vi "Begin.vi"(8 "error in":errorcluster) -> (0 "error out":errorcluster)   [LabVIEW 2017]
doc: "Called before other user functions, this VI is expected to open initial I/O refnums, load in file data, and do all program initialization. Notice that the <B>error out</B> terminal is simply used for data flow. Wiring it to other structures or subVIs ensures that this VI runs first."
uses:
  <vilib>/Rock Robotics/WPI/DriverStation/WPI_DriverStationRobotMode2.ctl
  <vilib>/Rock Robotics/WPI/Joystick/WPI_JoystickDeviceEnum.ctl
  <vilib>/Rock Robotics/WPI/ThirdParty/Phoenix-LabVIEW/Motor Controller/Controls/CTRE_Phoenix_MotorControl_ControlMode.ctl
  <vilib>/Rock Robotics/WPI/ThirdParty/Phoenix-LabVIEW/Motor Controller/Controls/CTRE_Phoenix_MotorControl_NeutralMode.ctl
  <vilib>/Rock Robotics/WPI/ThirdParty/Phoenix-LabVIEW/Motor Controller/Controls/CTRE_Phoenix_MotorControl_FeedbackDevice.ctl
  <vilib>/Rock Robotics/SystemInterfaces/spilib/spi_bus.ctl
  <vilib>/Rock Robotics/WPI/Solenoid/WPI_SolenoidChannel.ctl
  <vilib>/Rock Robotics/SystemInterfaces/DIO/FPGA_DIOChannel.ctl
  Robot Global Data.vi
  <vilib>/Rock Robotics/Network Tables/NT Write Numeric Array.vi
  <vilib>/Rock Robotics/WPI/Utilities/WPI_GetSetVariantRefNum.vi
  <vilib>/Rock Robotics/WPI/Gyro/WPI_GyroXRS450_SPI_Open.vi
  <vilib>/Rock Robotics/WPI/Switch/WPI_SwitchOpenLimit.vi
  <vilib>/Rock Robotics/WPI/Solenoid/WPI_SolenoidOpenDouble.vi
  <vilib>/Rock Robotics/Network Tables/NT Write String Array.vi
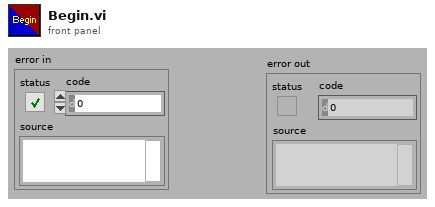
[diagram p1: front panel]
types:
  T1 = typedef "WPI_SolenoidChannel.ctl" = enum8{"Solenoid 0", "Solenoid 1", "Solenoid 2", "Solenoid 3", "Solenoid 4", "Solenoid 5", "Solenoid 6", "Solenoid 7", "Invalid"}
  T2 = typedef "FPGA_DIOChannel.ctl" = enum8{"DIO 0", "DIO 1", "DIO 2", "DIO 3", "DIO 4", "DIO 5", "DIO 6", "DIO 7", "DIO 8", "DIO 9", "DIO MXP 0", "DIO MXP 1", "DIO MXP 2", "DIO MXP 3", "DIO MXP 4", "DIO MXP 5", "DIO MXP 6", "DIO MXP 7", "DIO MXP 8", "DIO MXP 9", "DIO MXP 10", "DIO MXP 11", "DIO MXP 12", "DIO MXP 13", "DIO MXP 14", "DIO MXP 15", "SPI Port CS1", "SPI Port CS2", "SPI Port CS3", "SPI Port MISO", "SPI Port MOSI", "Invalid"}
  T3 = typedef "spi_bus.ctl" = enum16{"SPI On-Board, CS0", "SPI On-Board, CS1", "SPI On-Board, CS2", "SPI On-Board, CS3", "SPI MXP", "Invalid"}
  T4 = typedef "CTRE_Phoenix_MotorControl_FeedbackDevice.ctl" = i8
  T5 = typedef "CTRE_Phoenix_MotorControl_NeutralMode.ctl" = enum8{"EEPROMSetting", "Override to Coast", "Override to Brake"}
  T6 = typedef "CTRE_Phoenix_MotorControl_ControlMode.ctl" = u16
  T7 = typedef "WPI_JoystickDeviceEnum.ctl" = enum16{"USB 0", "USB 1", "USB 2", "USB 3", "USB 4", "USB 5"}
  T8 = typedef "WPI_DriverStationRobotMode2.ctl" = enum16{"Autonomous Disabled", "Autonomous Enabled", "Teleop Disabled", "Teleop Enabled", "Disconnected", "Finish", "Test Disabled", "Test Enabled", "Emergency Stopped"}
  T9 = typedef "WPI_SolenoidDevRef.ctl" = cluster{"DevStatus":errorcluster, "Pneumatics Control Module":u8, "Forward Solenoid Channel":T1, "Reverse Solenoid Channel":T1}
  T10 = typedef "WPI_JoystickDevRef.ctl" = cluster{"Device":T7}
  T11 = typedef "WPI_SwitchDevRef.ctl" = cluster{"DevStatus":errorcluster, "DIO Channel":T2, "CntIndex":T12, "Normally Closed":bool}
  T12 = typedef "FPGA_CounterCtrSystemIndex.ctl" = enum8{"Ctr 0", "Ctr 1", "Ctr 2", "Ctr 3", "Ctr 4", "Ctr 5", "Ctr 6", "Ctr 7", "Invalid"}
  T13 = typedef "WPI_MotorControlDeviceRef.ctl" = cluster{"DeviceStatus":errorcluster, "Type":T14, "PWM":cluster{"PWM Channel":T15, "DeadBand":T16}, "CAN":cluster{"Device Number":u8, "SetOutput VI Ref":variant, "GetOutput VI Ref":variant, "Enable VI Ref":variant, "Disable VI Ref":variant, "Data":variant}, "Invert":bool, "DIO PWM":cluster{"PWM \"Enable\" Channel":T15, "DIOChannel":T2, "PWM Rate":dbl}}
  T14 = typedef "WPI_MotorControlType.ctl" = enum16{"PWM", "CAN", "DIO PWM"}
  T15 = typedef "FPGA_DIOPWMChannel.ctl" = enum8{"PWM 0", "PWM 1", "PWM 2", "PWM 3", "PWM 4", "PWM 5", "PWM 6", "PWM 7", "PWM 8", "PWM 9", "PWM MXP 0", "PWM MXP 1", "PWM MXP 2", "PWM MXP 3", "PWM MXP 4", "PWM MXP 5", "PWM MXP 6", "PWM MXP 7", "PWM MXP 8", "PWM MXP 9", "Invalid"}
  T16 = typedef "WPI_PWMDeadband.ctl" = cluster{"Name":string, "maxPositivePwm":i32, "minPositivePwm":i32, "centerPwm":i32, "maxNegativePwm":i32, "minNegativePwm":i32, "angularRange":u16}
  T17 = typedef "WPI_GyroDevRef.ctl" = cluster{"DevStatus":errorcluster, "Analog Channel":T18, "Gain (VoltsPerDegree/Second)":dbl, "Gyro Type":enum16{"Analog", "XRS450"}, "Handle":i32, "SPI Bus":T3, "Device Found":bool, "Sample Rate":dbl, "Calibrate On Open":bool, "Offset":dbl}
  T18 = typedef "FPGA_AIChannel.ctl" = enum8{"AI 0", "AI 1", "AI 2", "AI 3", "AI MXP 0", "AI MXP 1", "AI MXP 2", "AI MXP 3", "Invalid"}
  T19 = typedef "WPI_CompressorDevRef.ctl" = cluster{"DevStatus":errorcluster, "Pneumatics Control Module":u8}
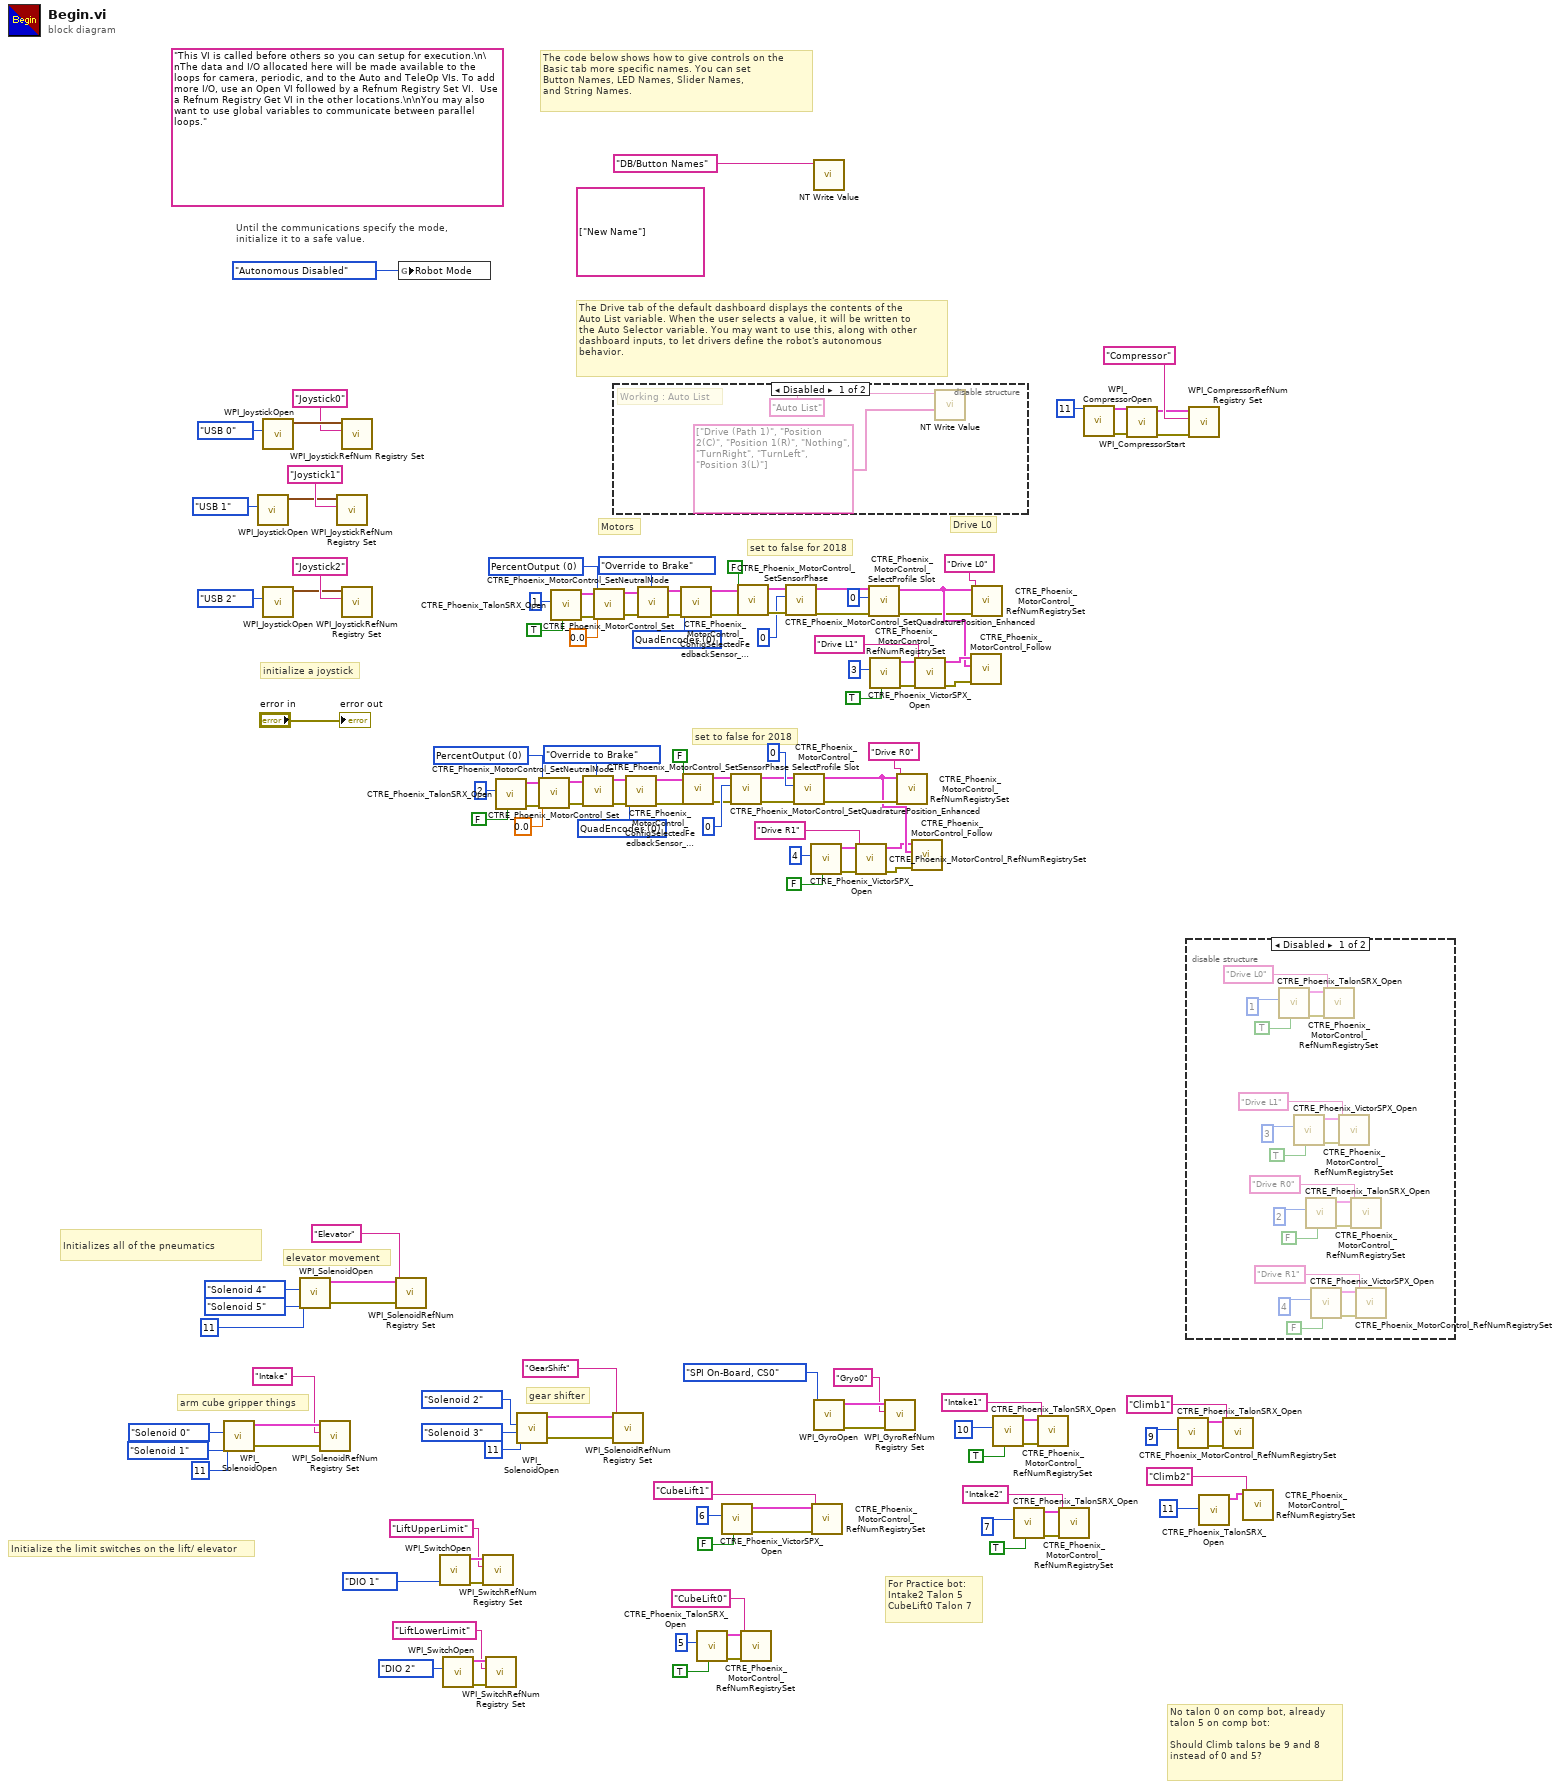
[diagram p0: block diagram]
diagram:
  w87 = T4 0 items=["None"=-1, "QuadEncoder"=0, "Analog"=2, "Tachometer"=4, "Pulse Width Encoded Position"=8, "Sensor Sum (S0 + S1)"=9, "Sensor Difference (D0 - D1)"=10, "Remote Source 0"=11, "Remote Source 1"=12, "Software Emulated"=15] ("Feedback Device")
  w82 = T6 0 items=["PercentOutput"=0, "Position"=1, "Velocity"=2, "Current"=3, "Follower"=5, "MotionProfile"=6, "MotionMagic"=7, "MotionMagicArc"=8, "MotionProfileArc"=10, "Disabled"=15] ("Control Mode")
  w106 = T4 0 items=["None"=-1, "QuadEncoder"=0, "Analog"=2, "Tachometer"=4, "Pulse Width Encoded Position"=8, "Sensor Sum (S0 + S1)"=9, "Sensor Difference (D0 - D1)"=10, "Remote Source 0"=11, "Remote Source 1"=12, "Software Emulated"=15] ("Feedback Device")
  w111 = T6 0 items=["PercentOutput"=0, "Position"=1, "Velocity"=2, "Current"=3, "Follower"=5, "MotionProfile"=6, "MotionMagic"=7, "MotionMagicArc"=8, "MotionProfileArc"=10, "Disabled"=15] ("Control Mode")
  (unwired) string[] ["New Name"]
  (unwired) "This VI is called before others so you can setup for execution.\n\nThe data and I/O allocated here will be made available to the loops for camera, periodic, and to the Auto and TeleOp VIs. To add more I/O, use an Open VI followed by a Refnum Registry Set VI.  Use a Refnum Registry Get VI in the other locations.\n\nYou may also want to use global variables to communicate between parallel loops."
  # "No talon 0 on comp bot, already\ntalon 5 on comp bot:\n\nShould Climb talons be 9 and 8\ninstead of 0 and 5?"
  # "gear shifter"
  # "arm cube gripper things"
  # "elevator movement"
  # "Initialize the limit switches on the lift/ elevator"
  # "Initializes all of the pneumatics"
  # "For Practice bot:\nIntake2 Talon 5\nCubeLift0 Talon 7"
  # "set to false for 2018"
  # "set to false for 2018"
  # "Drive L0"
  # "Motors"
  # "The Drive tab of the default dashboard displays the contents of the\nAuto List variable. When the user selects a value, it will be written to\nthe Auto Selector variable. You may want to use this, along with other\ndashboard inputs, to let drivers define the robot's autonomous\nbehavior."
  # "The code below shows how to give controls on the\nBasic tab more specific names. You can set\nButton Names, LED Names, Slider Names,\nand String Names."
  # "initialize a joystick"
  # "Until the communications specify the mode,\ninitialize it to a safe value."
  n1 = call-poly <vilib>:"WPI_SolenoidOpen.vi"("Reverse Solenoid Channel"=WPI_SolenoidChannel."Solenoid 1", "Forward Solenoid Channel"=WPI_SolenoidChannel."Solenoid 0", "Pneumatics Control Module (0)"=u8 11) -> ("error out"=w24:errorcluster, "SolenoidDevRef"=w23:T9)  [unwired: 7 in]
  n2 = call <vilib>:"WPI_JoystickOpen.vi"("JoystickDevice"=WPI_JoystickDeviceEnum."USB 1") -> ("JoystickDevRef"=w135:T10)  [unwired: 10 in]
  n3 = call <vilib>:"WPI_JoystickOpen.vi"("JoystickDevice"=WPI_JoystickDeviceEnum."USB 0") -> ("JoystickDevRef"=w130:T10)  [unwired: 10 in]
  n4 = call <vilib>:"WPI_JoystickOpen.vi"("JoystickDevice"=WPI_JoystickDeviceEnum."USB 2") -> ("JoystickDevRef"=w127:T10)  [unwired: 10 in]
  n5 = call-poly <vilib>:"WPI_SolenoidOpen.vi"("Reverse Solenoid Channel"=WPI_SolenoidChannel."Solenoid 5", "Forward Solenoid Channel"=WPI_SolenoidChannel."Solenoid 4", "Pneumatics Control Module (0)"=u8 11) -> ("error out"=w32:errorcluster, "SolenoidDevRef"=w31:T9)  [unwired: 7 in]
  n6 = call <vilib>:"WPI_SolenoidRefNum Registry Set.vi"("error in (no error)"=w24, "refnum name"="Intake", "SolenoidDevRef"=w23) -> ()  [unwired: 7 in, 2 out]
  n7 = call <vilib>:"WPI_JoystickRefNum Registry Set.vi"("refnum name"="Joystick1", "JoystickDevRef"=w135) -> ()  [unwired: 8 in, 2 out]
  n8 = call <vilib>:"WPI_JoystickRefNum Registry Set.vi"("refnum name"="Joystick0", "JoystickDevRef"=w130) -> ()  [unwired: 8 in, 2 out]
  n9 = call <vilib>:"WPI_JoystickRefNum Registry Set.vi"("refnum name"="Joystick2", "JoystickDevRef"=w127) -> ()  [unwired: 8 in, 2 out]
  n10 = call <vilib>:"WPI_SolenoidRefNum Registry Set.vi"("error in (no error)"=w32, "refnum name"="Elevator", "SolenoidDevRef"=w31) -> ()  [unwired: 7 in, 2 out]
  n11 = global write "Robot Global Data.vi" "Robot Mode"(WPI_DriverStationRobotMode2."Autonomous Disabled" ("Robot Mode")) -> ()
  n12 = call-poly <vilib>:"WPI_SwitchOpen.vi"("DIO Channel"=FPGA_DIOChannel."DIO 1") -> ("error out"=w20:errorcluster, "SwitchDevRef"=w19:T11)  [unwired: 9 in]
  n13 = call-poly <vilib>:"WPI_SwitchOpen.vi"("DIO Channel"=FPGA_DIOChannel."DIO 2") -> ("error out"=w17:errorcluster, "SwitchDevRef"=w16:T11)  [unwired: 9 in]
  n14 = call <vilib>:"WPI_SwitchRefNum Registry Set.vi"("error in (no error)"=w20, "refnum name"="LiftUpperLimit", "SwitchDevRef"=w19) -> ()  [unwired: 7 in, 2 out]
  n15 = call <vilib>:"WPI_SwitchRefNum Registry Set.vi"("error in (no error)"=w17, "refnum name"="LiftLowerLimit", "SwitchDevRef"=w16) -> ()  [unwired: 7 in, 2 out]
  n16 = call "CTRE_Phoenix_TalonSRX_Open.vi"("Invert"=FALSE, "Device Number"=u8 2) -> ("error out"=w79:errorcluster, "CAN Talon SRX Ref"=w78:T13)  [unwired: 8 in]
  n17 = call-poly <vilib>:"WPI_SolenoidOpen.vi"("Reverse Solenoid Channel"=WPI_SolenoidChannel."Solenoid 3", "Forward Solenoid Channel"=WPI_SolenoidChannel."Solenoid 2", "Pneumatics Control Module (0)"=u8 11) -> ("error out"=w25:errorcluster, "SolenoidDevRef"=w26:T9)  [unwired: 7 in]
  n18 = call <vilib>:"CTRE_Phoenix_MotorControl_Set.vi"("error in (no error)"=w79, "Output"=0.0, "Control Mode"=w82, "PhoenixMotorControlDevRef"=w78) -> ("error out"=w81:errorcluster, "PhoenixMotorControlDevRef"=w80:T13)  [unwired: 6 in]
  n19 = call "CTRE_Phoenix_TalonSRX_Open.vi"("Invert"=TRUE, "Device Number"=u8 1) -> ("error out"=w114:errorcluster, "CAN Talon SRX Ref"=w115:T13)  [unwired: 8 in]
  n20 = call <vilib>:"CTRE_Phoenix_MotorControl_SetNeutralMode.vi"("error in (no error)"=w81, "Motor Control Neutral Mode"=CTRE_Phoenix_MotorControl_NeutralMode."Override to Brake", "PhoenixMotorControlDevRef"=w80) -> ("error out"=w85:errorcluster, "PhoenixMotorControlDevRef"=w86:T13)  [unwired: 7 in]
  n21 = call <vilib>:"CTRE_Phoenix_MotorControl_Set.vi"("error in (no error)"=w114, "Output"=0.0, "Control Mode"=w111, "PhoenixMotorControlDevRef"=w115) -> ("error out"=w112:errorcluster, "PhoenixMotorControlDevRef"=w113:T13)  [unwired: 6 in]
  n22 = call <vilib>:"WPI_SolenoidRefNum Registry Set.vi"("error in (no error)"=w25, "refnum name"="GearShift", "SolenoidDevRef"=w26) -> ()  [unwired: 7 in, 2 out]
  n23 = disable-structure shown="Disabled" {
    frame Disabled {
      # "Working : Auto List"
      n24 = call-poly <vilib>:"NT Write Value.vi"("String Array"=string[] ["Drive (Path 1)", "Position 2(C)", "Position 1(R)", "Nothing", "TurnRight", "TurnLeft", "Position 3(L)"], "Name"="Auto List") -> ()  [unwired: 9 in, 1 out]
    }
    frame Enabled {
    }
  }
  n25 = call <vilib>:"CTRE_Phoenix_MotorControl_ConfigSelectedFeedbackSensor_Enhanced.vi"("error in (no error)"=w85, "Feedback Device"=w87, "PhoenixMotorControlDevRef"=w86) -> ("error out"=w89:errorcluster, "PhoenixMotorControlDevRef"=w88:T13)  [unwired: 7 in]
  n26 = call <vilib>:"CTRE_Phoenix_MotorControl_SetNeutralMode.vi"("error in (no error)"=w112, "Motor Control Neutral Mode"=CTRE_Phoenix_MotorControl_NeutralMode."Override to Brake", "PhoenixMotorControlDevRef"=w113) -> ("error out"=w108:errorcluster, "PhoenixMotorControlDevRef"=w107:T13)  [unwired: 7 in]
  n27 = call <vilib>:"CTRE_Phoenix_MotorControl_ConfigSelectedFeedbackSensor_Enhanced.vi"("error in (no error)"=w108, "Feedback Device"=w106, "PhoenixMotorControlDevRef"=w107) -> ("error out"=w104:errorcluster, "PhoenixMotorControlDevRef"=w105:T13)  [unwired: 7 in]
  n28 = call <vilib>:"CTRE_Phoenix_MotorControl_SetSensorPhase.vi"("error in (no error)"=w89, "PhaseSensor"=FALSE, "PhoenixMotorControlDevRef"=w88) -> ("error out"=w91:errorcluster, "PhoenixMotorControlDevRef"=w92:T13)  [unwired: 7 in]
  n29 = call "CTRE_Phoenix_TalonSRX_Open.vi"("Invert"=TRUE, "Device Number"=u8 5) -> ("error out"=w44:errorcluster, "CAN Talon SRX Ref"=w43:T13)  [unwired: 8 in]
  n30 = call <vilib>:"CTRE_Phoenix_VictorSPX_Open.vi"("Invert"=FALSE, "Device Number"=u8 6) -> ("error out"=w47:errorcluster, "CAN Talon SRX Ref"=w46:T13)  [unwired: 8 in]
  n31 = call <vilib>:"CTRE_Phoenix_MotorControl_SetQuadraturePosition_Enhanced.vi"("error in (no error)"=w91, "New Position"=0, "PhoenixMotorControlDevRef"=w92) -> ("error out"=w3:errorcluster, "PhoenixMotorControlDevRef"=w4:T13)  [unwired: 7 in]
  n32 = call <vilib>:"CTRE_Phoenix_MotorControl_SetSensorPhase.vi"("error in (no error)"=w104, "PhaseSensor"=FALSE, "PhoenixMotorControlDevRef"=w105) -> ("error out"=w102:errorcluster, "PhoenixMotorControlDevRef"=w101:T13)  [unwired: 7 in]
  n33 = call <vilib>:"CTRE_Phoenix_MotorControl_RefNumRegistrySet.vi"("error in (no error)"=w44, "refnum name"="CubeLift0", "PhoenixMotorControlDevRef"=w43) -> ()  [unwired: 7 in, 2 out]
  n34 = call <vilib>:"CTRE_Phoenix_MotorControl_SetQuadraturePosition_Enhanced.vi"("error in (no error)"=w102, "New Position"=0, "PhoenixMotorControlDevRef"=w101) -> ("error out"=w5:errorcluster, "PhoenixMotorControlDevRef"=w6:T13)  [unwired: 7 in]
  n35 = call <vilib>:"CTRE_Phoenix_MotorControl_SelectProfile Slot.vi"("error in (no error)"=w3, "slotIdx"=0, "PhoenixMotorControlDevRef"=w4) -> ("error out"=w95:errorcluster, "PhoenixMotorControlDevRef"=w94:T13)  [unwired: 7 in]
  n36 = call <vilib>:"CTRE_Phoenix_VictorSPX_Open.vi"("Invert"=FALSE, "Device Number"=u8 4) -> ("error out"=w71:errorcluster, "CAN Talon SRX Ref"=w72:T13)  [unwired: 8 in]
  n37 = call <vilib>:"CTRE_Phoenix_MotorControl_RefNumRegistrySet.vi"("error in (no error)"=w47, "refnum name"="CubeLift1", "PhoenixMotorControlDevRef"=w46) -> ()  [unwired: 7 in, 2 out]
  n38 = call-poly <vilib>:"NT Write Value.vi"("Name"="DB/Button Names") -> ()  [unwired: 10 in, 1 out]
  n39 = call-poly <vilib>:"WPI_GyroOpen.vi"("SPI Bus"=spi_bus."SPI On-Board, CS0") -> ("error out"=w39:errorcluster, "GyroDevRef"=w40:T17)  [unwired: 8 in, 1 out]
  n40 = call <vilib>:"CTRE_Phoenix_MotorControl_RefNumRegistrySet.vi"("error in (no error)"=w71, "refnum name"="Drive R1", "PhoenixMotorControlDevRef"=w72) -> ("error out"=w74:errorcluster, "PhoenixMotorControlDevRef"=w75:T13)  [unwired: 7 in]
  n41 = call <vilib>:"CTRE_Phoenix_MotorControl_SelectProfile Slot.vi"("error in (no error)"=w5, "slotIdx"=0, "PhoenixMotorControlDevRef"=w6) -> ("error out"=w98:errorcluster, "PhoenixMotorControlDevRef"=w99:T13)  [unwired: 7 in]
  n42 = call <vilib>:"CTRE_Phoenix_VictorSPX_Open.vi"("Invert"=TRUE, "Device Number"=u8 3) -> ("error out"=w122:errorcluster, "CAN Talon SRX Ref"=w121:T13)  [unwired: 8 in]
  n43 = call <vilib>:"WPI_GyroRefNum Registry Set.vi"("error in (no error)"=w39, "refnum name"="Gryo0", "GyroDevRef"=w40) -> ()  [unwired: 7 in, 2 out]
  n44 = call <vilib>:"CTRE_Phoenix_MotorControl_RefNumRegistrySet.vi"("error in (no error)"=w95, "refnum name"="Drive R0", "PhoenixMotorControlDevRef"=w94) -> ()  [unwired: 7 in, 2 out]
  n45 = call <vilib>:"CTRE_Phoenix_MotorControl_Follow.vi"("error in (no error)"=w74, "Master Controller to Follow"=w94, "PhoenixMotorControlDevRef"=w75) -> ()  [unwired: 7 in, 2 out]
  n46 = call <vilib>:"CTRE_Phoenix_MotorControl_RefNumRegistrySet.vi"("error in (no error)"=w122, "refnum name"="Drive L1", "PhoenixMotorControlDevRef"=w121) -> ("error out"=w119:errorcluster, "PhoenixMotorControlDevRef"=w118:T13)  [unwired: 7 in]
  n47 = call <vilib>:"CTRE_Phoenix_MotorControl_Follow.vi"("error in (no error)"=w119, "Master Controller to Follow"=w99, "PhoenixMotorControlDevRef"=w118) -> ()  [unwired: 7 in, 2 out]
  n48 = call <vilib>:"CTRE_Phoenix_MotorControl_RefNumRegistrySet.vi"("error in (no error)"=w98, "refnum name"="Drive L0", "PhoenixMotorControlDevRef"=w99) -> ()  [unwired: 7 in, 2 out]
  n49 = call "CTRE_Phoenix_TalonSRX_Open.vi"("Invert"=TRUE, "Device Number"=u8 10) -> ("error out"=w56:errorcluster, "CAN Talon SRX Ref"=w55:T13)  [unwired: 8 in]
  n50 = call "CTRE_Phoenix_TalonSRX_Open.vi"("Invert"=TRUE, "Device Number"=u8 7) -> ("error out"=w52:errorcluster, "CAN Talon SRX Ref"=w51:T13)  [unwired: 8 in]
  n51 = call <vilib>:"CTRE_Phoenix_MotorControl_RefNumRegistrySet.vi"("error in (no error)"=w56, "refnum name"="Intake1", "PhoenixMotorControlDevRef"=w55) -> ()  [unwired: 7 in, 2 out]
  n52 = call <vilib>:"CTRE_Phoenix_MotorControl_RefNumRegistrySet.vi"("error in (no error)"=w52, "refnum name"="Intake2", "PhoenixMotorControlDevRef"=w51) -> ()  [unwired: 7 in, 2 out]
  n53 = call <vilib>:"WPI_CompressorOpen.vi"("Pneumatics Control Module (0)"=u8 11) -> ("CompressorDevRef"=w66:T19, "error out"=w65:errorcluster)  [unwired: 13 in]
  n54 = call <vilib>:"WPI_CompressorStart.vi"("error in (no error)"=w65, "CompressorDevRef"=w66) -> ("error out"=w63:errorcluster, "CompressorDevRef"=w64:T19)  [unwired: 8 in]
  n55 = call "CTRE_Phoenix_TalonSRX_Open.vi"("Device Number"=u8 9) -> ("error out"=w61:errorcluster, "CAN Talon SRX Ref"=w60:T13)  [unwired: 9 in]
  n56 = disable-structure shown="Disabled" {
    frame Disabled {
      n57 = call "CTRE_Phoenix_TalonSRX_Open.vi"("Invert"=TRUE, "Device Number"=u8 1) -> ("error out"=w156:errorcluster, "CAN Talon SRX Ref"=w157:T13)  [unwired: 8 in]
      n58 = call <vilib>:"CTRE_Phoenix_VictorSPX_Open.vi"("Invert"=TRUE, "Device Number"=u8 3) -> ("error out"=w155:errorcluster, "CAN Talon SRX Ref"=w154:T13)  [unwired: 8 in]
      n59 = call "CTRE_Phoenix_TalonSRX_Open.vi"("Invert"=FALSE, "Device Number"=u8 2) -> ("error out"=w148:errorcluster, "CAN Talon SRX Ref"=w149:T13)  [unwired: 8 in]
      n60 = call <vilib>:"CTRE_Phoenix_VictorSPX_Open.vi"("Invert"=FALSE, "Device Number"=u8 4) -> ("error out"=w147:errorcluster, "CAN Talon SRX Ref"=w146:T13)  [unwired: 8 in]
      n61 = call <vilib>:"CTRE_Phoenix_MotorControl_RefNumRegistrySet.vi"("error in (no error)"=w156, "refnum name"="Drive L0", "PhoenixMotorControlDevRef"=w157) -> ()  [unwired: 7 in, 2 out]
      n62 = call <vilib>:"CTRE_Phoenix_MotorControl_RefNumRegistrySet.vi"("error in (no error)"=w155, "refnum name"="Drive L1", "PhoenixMotorControlDevRef"=w154) -> ()  [unwired: 7 in, 2 out]
      n63 = call <vilib>:"CTRE_Phoenix_MotorControl_RefNumRegistrySet.vi"("error in (no error)"=w148, "refnum name"="Drive R0", "PhoenixMotorControlDevRef"=w149) -> ()  [unwired: 7 in, 2 out]
      n64 = call <vilib>:"CTRE_Phoenix_MotorControl_RefNumRegistrySet.vi"("error in (no error)"=w147, "refnum name"="Drive R1", "PhoenixMotorControlDevRef"=w146) -> ()  [unwired: 7 in, 2 out]
    }
    frame Enabled {
    }
  }
  n65 = call <vilib>:"WPI_CompressorRefNum Registry Set.vi"("error in (no error)"=w63, "refnum name"="Compressor", "CompressorDevRef"=w64) -> ()  [unwired: 7 in, 2 out]
  n66 = call "CTRE_Phoenix_TalonSRX_Open.vi"("Device Number"=u8 11) -> ("CAN Talon SRX Ref"=w1:T13)  [unwired: 9 in, 1 out]
  n67 = call <vilib>:"CTRE_Phoenix_MotorControl_RefNumRegistrySet.vi"("error in (no error)"=w61, "refnum name"="Climb1", "PhoenixMotorControlDevRef"=w60) -> ()  [unwired: 7 in, 2 out]
  n68 = call <vilib>:"CTRE_Phoenix_MotorControl_RefNumRegistrySet.vi"("refnum name"="Climb2", "PhoenixMotorControlDevRef"=w1) -> ()  [unwired: 8 in, 2 out]
  "error out" <- "error in"
